vi "Create Transfer Group Timing.vi"(11 "Transfer Groups":refnum<class "Transfer Group.lvclass">[](array[class])) -> (3 "Transfer Group Timings":refnum<class "Transfer Group Timing.lvclass">[](array[class]))   [LabVIEW 2017, in "DSF Core.lvlib" / "Scheduler.lvclass"]
uses:
  Scheduler.lvclass
  Timing/Transfer Group Timing.lvclass
  Transfer Group/Transfer Group.lvclass
  Transfer Group/Transfer Group.lvclass/Transfer Group.ctl
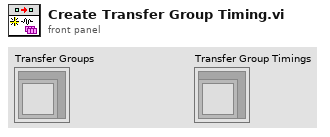
[diagram p1: front panel]
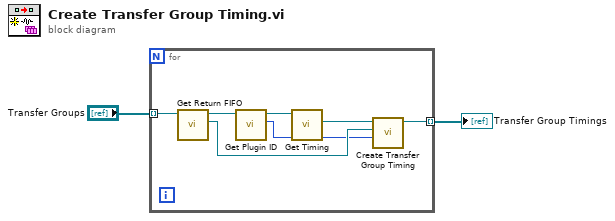
[diagram p0: block diagram]
diagram:
  n1 = for {
    tunnel: "Transfer Groups" -> [w8] mode=indexing
    tunnel: [w3] -> w1 mode=indexing
    n2 = call "Get Return FIFO.vi"("Transfer Group in"=w8) -> ("Return FIFO"=w5:refnum<k33>, "Transfer Group out"=w7:refnum<class "Transfer Group.lvclass">)  [unwired: 9 in]
    n3 = call "Get Plugin ID.vi"("Transfer Group in"=w7) -> ("plugin id"=w4:i32, "Transfer Group out"=w9:refnum<class "Transfer Group.lvclass">)  [unwired: 9 in]
    n4 = call "Get Timing.vi"("Transfer Group in"=w9) -> ("Timing"=w6:refnum<class "Timing.lvclass">)  [unwired: 9 in, 1 out]
    n5 = call "Create Transfer Group Timing.vi"("ID"=w4, "Return FIFO"=w5, "Timing"=w6) -> ("Transfer Group Timing out"=w3:refnum<class "Transfer Group Timing.lvclass">)  [unwired: 7 in, 1 out]
  }
  "Transfer Group Timings" <- w1
